vi "xwav2xy.vi"   [LabVIEW 2015]
uses:
  _xwav_polys.lvlib
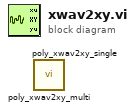
[diagram p0: block diagram]
diagram:
  n1 = call "poly_xwav2xy_multi.vi"() -> ()  [unwired: 7 in, 5 out]
  n2 = call "poly_xwav2xy_single.vi"() -> ()  [unwired: 7 in, 5 out]
